vi "table_background_color.vi"() -> ()   [LabVIEW 2021]
panel:
  in  "Table Control":string[][](table)
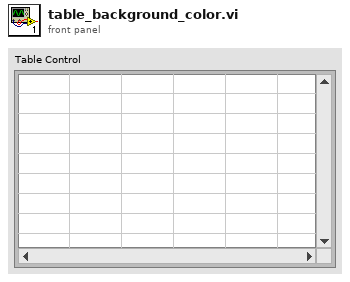
[diagram p1: front panel]
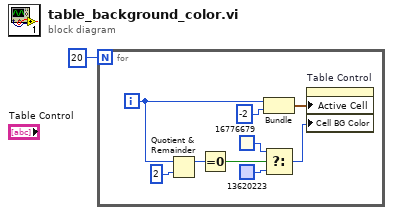
[diagram p0: block diagram]
diagram:
  n1 = for {
    N: 20 -> [_]
    i -> [w8]
    n2 = Quotient & Remainder(x=w8, y=2) -> (x-y*floor(x/y)=w6:i32)  [unwired: 1 out]
    n3 = Equal To 0?(x=w6) -> (x = 0?=w5:bool)
    n4 = Bundle(w8, -2) -> (w9:cluster{i32, i32})  [unwired: 1 in]
    n5 = Select(t=u32 16776679, s=w5, f=u32 13620223) -> (s? t:f=w2:u32)
    n6 = property on="Table Control" class="Tbl (strict)"("Active Cell"=w9, "Cell BG Color"=w2) -> ()  [unwired: 2 in, 2 out]
  }
